vi "4_1_2.vi"() -> ()   [LabVIEW 2023, in "2025.lvlib"]
uses:
  2025.lvlib
  Program Files/National Instruments/LabVIEW 2025/user.lib/_OpenG.lib/lvdata/lvdata.llb/openg_variant.lvlib
panel:
  out "Intensity Graph":i32[][](graph)
  out "Array 3":i32[][](array[numeric])
  in  "Boolean":bool
  out "Result":i32
  out "Array 2":i32[](array[numeric])
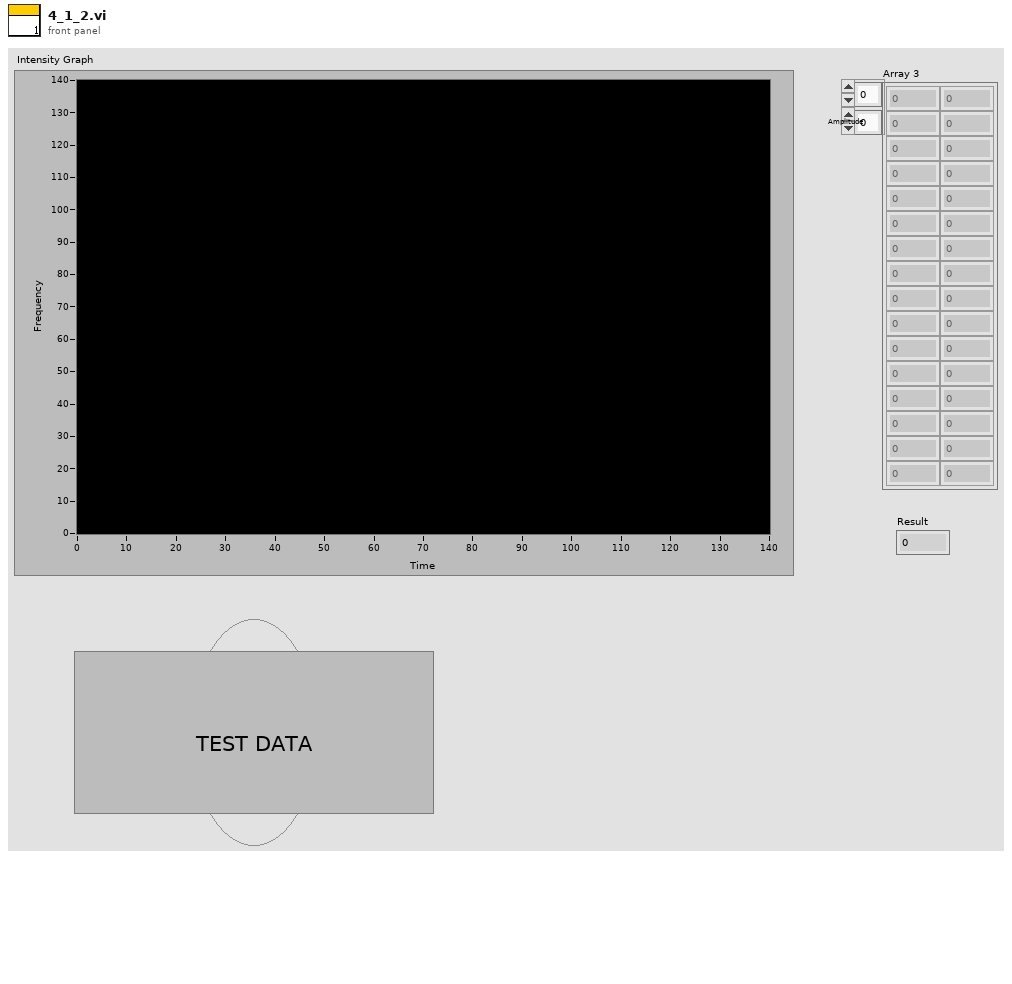
[diagram p1: front panel]
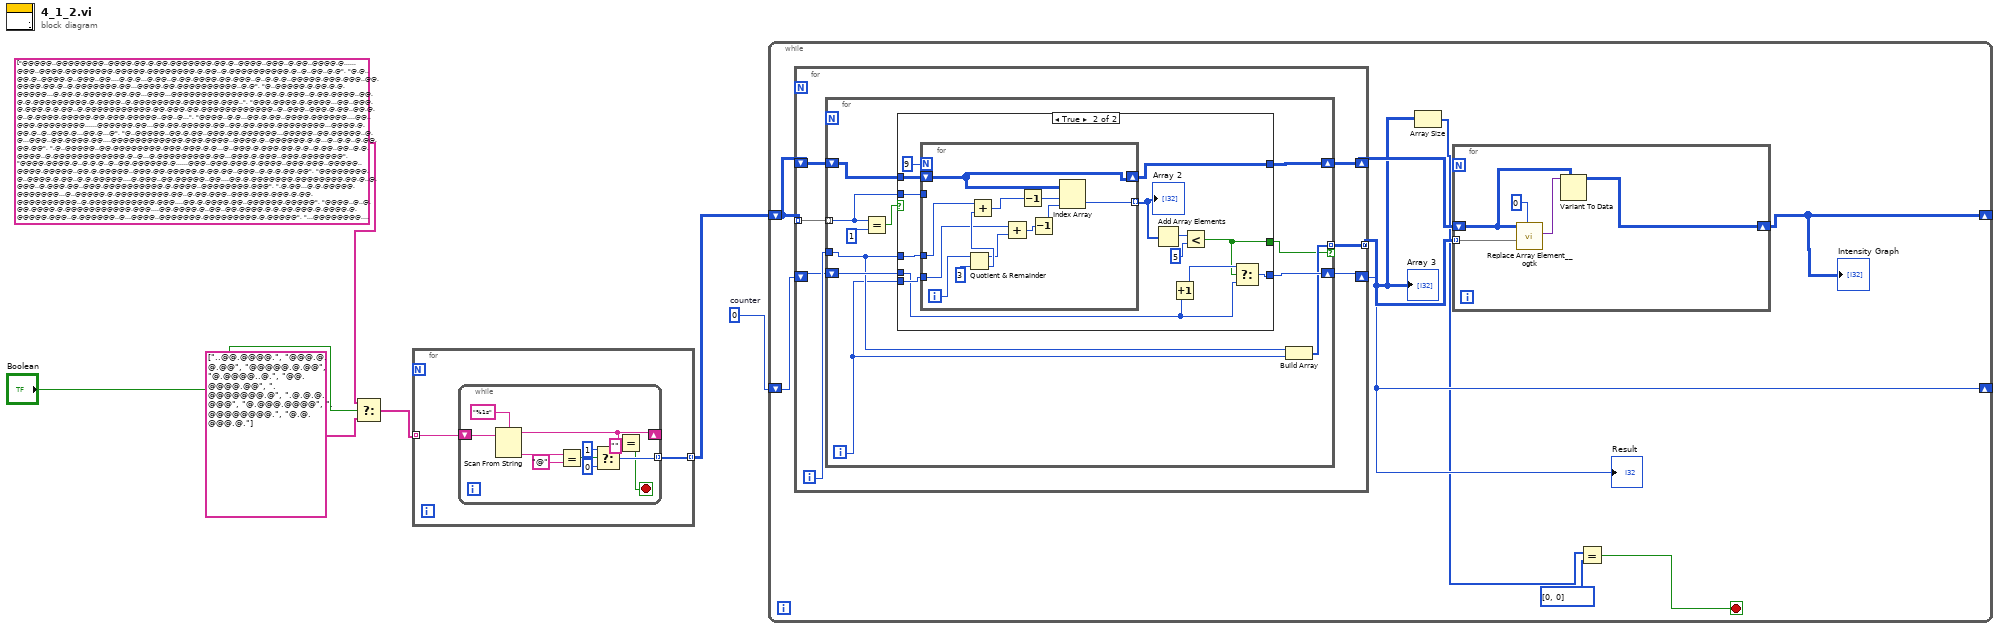
[diagram p0: block diagram]
diagram:
  w5 = 0  # counter
  n1 = Select(t=string[] ["@@@@@..@@@@@@@@..@@@@.@@.@.@@.@@@@@@@.@@.@..@@@@..@@@..@.@@..@@@@.@......@@@..@@@@.@@@@@@@@.@@@@@.@@@@@@@@.@.@@..@.@@@@@@@@@@.@..@..@@..@.@", "@.@..@@.@..@@@@.@..@@@..@@....@.@.@...@.@@..@.@@.@@@@.@@.@@@..@..@.@.@..@@@@@.@@@.@@@..@@.@@@@.@@.@..@.@@@@@@@.@@...@@@@.@@.@@@@@@@@@@..@.@", "@..@@@@@.@.@@.@.@.@@@@@...@.@@.@.@@@@@.@@.@@...@@@...@@@@@@@@@@@@@@.@.@@.@.@@@..@.@@.@@@@..@@.@.@.@@@@@@@@@.@.@@@@..@.@@@@@@@@.@@@@@@.@@@..", "@@@.@@@@.@.@@@@...@@..@@@.@.@@@.@.@.@@..@.@@@@@@@@@@@.@@.@@@.@@.@@@@@@@@@@@@..@..@@@..@@@.@.@@..@@.@.@..@.@@@@.@@@@@.@@.@@@.@@@@@..@@..@...", "@@@@..@.@...@@.@.@@..@@@@.@@@@@@....@@..@@@.@@@@@@@@......@@@@@@.@@...@@.@@.@@@@@.@@..@@.@@.@@@.@@@@@@@@...@@@@.@.@@.@..@..@@@.@...@@.@...@", "@..@@@@@..@@.@.@@..@@@.@@.@@@@@@...@@@@@..@@.@@@@@..@.@...@@@..@@.@@@@.@@....@@@@@@@@@@@@.@@@.@@@@..@@@@.@..@@@@@@.@.@...@..@.@..@.@@.@@.@@", ".@..@@@@@..@@.@@@@@@@@.@@@.@@@.@.@...@..@@@.@.@@@.@@.@.@..@.@@..@@..@.@.@@@@..@.@@@@@@@@@@@@.@..@...@.@@@@@@@@@.@@...@@@.@.@@@..@@@.@@@@@@@", "@@@@.@@@@.@..@.@.@..@..@@.@@@@@@.@......@@@..@@@.@@@.@.@@@@..@@@.@@@..@@@@@..@@@@.@@@@@..@@.@.@@@@@..@@@.@@.@@@@@.@.@@.@@..@@@..@.@.@.@@.@@", "@@@@@@@@.@..@@@@.@.@@..@.@.@@@@@....@.@@@..@@.@@@@@..@@....@@.@.@@@@@@@.@@@@@@@@.@@.@..@.@@@..@.@@@.@@..@@@.@@@@@@@@@@.@.@@@@..@@@@@@@@.@@@", ".@.@@...@.@.@@@@@.@@@@@@@...@..@@@@@.@.@@@@@@@@@.@@..@.@@.@@@..@@@.@@@.@@@.@.@@.@@@@@@@@@@..@.@@@@@@@@@@@.@@@....@@.@.@@@@.@@..@@@@@@.@@@@@", "@@@@..@..@.@@.@@@@.@.@@@@@@@@@@@.@@@....@@.@@@@.@..@@..@@.@@@@.@.@.@@.@@@.@.@@@@.@.@@@@@.@@@..@.@@@@@@..@...@@@@..@@@@@@@.@@@@@@@@@.@.@@@@@", "...@@@@@@@@.@@@@...@@.@..@@@@@@@@@.@@@.@@@@.@@.@@....@@...@@@.@.@.@@@@@@@@@@.@@.@.@.@@@.@@..@@..@@.@.@.@.@.@.@@@@.@..@.@..@@@@.@.@@@@@.@@@.", "@@@...@@@@@..@.@.@...@@..@.@@@@..@@@@...@@@@.@@@@@.@@@@.@@@@@..@.@@@@@.@@@@.@@@.@@@@..@@@@@..@.@@@...@@...@@@@@@@@.@.@@@..@@.@@@.....@@.@@@", ".@@@@@.@@@@@@@..@@.@@@@@@@@@@.@@.@@.@@@@@.@@@@@..@@@@@@@@@..@@@@@@@@@.@@@..@.@.@@....@@..@..@.@@@.@@@@@@...@@@@@@@@@@@.@.@@..@.@@.@@@@.@@..", "..@@@@@@@@@@.@.@@@@@@.@..@@.@.@@@@@@@@.@.@@@@@@@@.@.@@@.@@@@.@@@..@@..@@@@@.@@@.@@@@@@.@@@..@@@@@...@@@.@@@.@.@@...@@.@@@.@@@@@@@@@@@@@@@@@", "@@.@..@@@.@@@.@@@@@@@@@@@..@..@.@@.@@@.@@@@@@@.@..@..@@@..@@@...@..@@@@@...@@.@@@@@@@@...@@..@@.@@@@....@@@@.....@.@...@@@..@@@@.@@@.@@@@@@", "@@..@@.@@@.@@@@..@.@@@.@@.@@@@@@.@..@@@@@...@@@@@@@..@.....@@.@@.@..@@@..@@@@.@@@..@.@.@@@@.@@@@@@@@@@@@@@@@.@@.@.@.@@@@.@@..@.@@...@..@.@@", "@@@.@@@@@@@@@@.@@@@.@@@@@@@@.@@@@@.@@@.@@..@.@@..@@@@@..@.@.....@.@@@@@..@.@@@.@@@@.@..@..@..@@@...@@@@..@.@.@@@@.@...@@@@@@@...@..@@.@@.@.", "@.@@...@@.@@@@@@@..@.@.@@@..@@.@.@@@@...@.@@@@@@@@@@@@@@@..@@@@.@@....@@@@@...@@.@@.@@@@@@.@@.@@.@@.@@.@@.@@@.@.@.@@@@.@@.@.@@..@@..@.@@@@@", "@@@@.@.@.@@@@@@@..@@@@@..@@.@.@@@.@@@.@.@@@@@@@@@@@@@@@@@...@@@....@.@.@@@@@@.@....@..@@.@@@@@..@@.@@@@@.@@@@.@@@@@..@@@@@.@@@@.@.@.@@@..@.", "@@@.@@.@@@.@@@@.@@.@@@.@..@@.@..@@@@@.....@.@@.@.@@.@@.@@@.@.@@@.@@.@@@@..@..@@@..@@@@@.@....@@..@.@@@@@.@.@@@@..@@@@@@@@.@@....@@.@@.@@@..", ".@@.@@.@@..@@@.@@@@@@@.@@@.@@@@@@@..@@.@@@.@@@@.@@.@..@@@.@@.....@.@@...@@.@.@@.@@@@@@@@.@@..@@@.@.@.@@.@@@@@@@.@..@@@@.@@@@@@@@..@..@@.@..", "@@@...@@@.@@@@.@.@@.@@..@@@@@@@@@@@@.@.@@.@..@@@@@.@@@...@@@.@@.@.@.@......@@.@@.@.@@@.@@@@@..@@.@.@@..@@@@@@@.@@@..@..@@...@@@@@@@@@@@@@.@", "@@@@.@....@@@@@@@@@@@..@@..@.@@..@@@@.@@@@@.@.@@@.@.@@.@@@@@@@@.@...@@.@@.@@@.@@@.@..@@.@@.@@..@@.@...@@@.@.@@@...@@@.@@@@@@@@.@.@@.@..@@@@", "@@@@.@.@.@@@@@@@@.@@@@@.@.@.@.@.@@.@@@.@@@.....@@.@.@.@@@.....@@..@.@@@@@.@...@@@@@@.@@@.@.@..@@.@@@@@...@@@@.@.@.@..@@@..@@@@@@.@@.@@@.@..", "..@@@.@.@@@@@@@@..@@@..@@@@@@@@@@.@.@@@@@@@@@..@@@@...@@@@.@..@@..@@@@.@@@@.@@@.@@.@@@@....@.@.@..@.@.@@..@@.@@@@@@.@...@@.@@@.@..@@@@.@.@@", "..@@@@@.@.@@@.@@..@.@..@.@@@@@@@@@.@...@..@@@@@.@@@@@.@...@@....@@@@@.@.@@.@.@.@.@.@.@@@@@@...@@..@...@@@@.@@@@.@.@..@.@@@@@@@@@@.@@@@.@.@@", ".@@@@@..@@@@.@@@@@..@@@.@@.@..@...@@@..@@@@@.@@.@@..@@@.@@..@@...@@@.@.@...@@.@@@@@..@@@@@.@@@@@@.@.@@@@.@.@.@.@@@@@.@@@@...@@@@@.@@@@@@.@.", "@@@.@@..@...@@@@@@..@@@@@@@...@@@@@@@@......@@.@@.@@.@.@.@.@@..@@..@@.@.@.@@.@@@.@@@@@@@@@@@.@@.@@..@@@@...@@@@@@@@.@.@@@.@.@@@..@@@@@@...@", "@..@@..@@@@@.@@@@.@.@@@.@..@.@.@.@.@@@.....@@@.@.@.@@.@@.@@..@@@@@@@@@...@@....@.@.@@@..@@..@@@@@...@@@@@@@@@@@@@@@@@@@.@...@@@@..@.@.@@@@@", "@@..@.@@@.@@@..@.@@.@@@@@@..@@.@..@@@@@@.@@@.@@@...@@.@.@@@@.@.@@@@@..@@@@@@.@@@@.@.@@@@@@@@@@..@@.@@.@@.@@@.@.@@@..@@.@@.@@.@.@@@@@@@..@..", "@..@@.@..@@@@@@@.@.@...@.@@@@@@.@@@@@....@@@@@....@@@.@@..@@@@..@@@.@.@@@@@@@@.@..@@@@@..@@@@@@@@.@@@.@@@@@@@@.@@@@.@@..@@...@@@@@.@@@.@@@.", "@@@@@@@..@@@.@..@.@..@@.@.@@@@.@@@@.....@@.@.@@@.@@..@@.@@@.@..@@.@.@@.@.@.@@.@@@.@@.@@.@@@@@.@..@@.@...@@.@..@@@@@@@@@..@@@@@.@@.@@..@.@.@", "@.@@@.@.@.@@.@@@@.@@....@@@@@.@@@..@..@@....@.@@@@@@..@@@.@@@@@@..@.@.@@@....@.@...@@@.@@@@@.@.@.@@@@@..@@@.@.@@..@@.@.@.@@@@@@.@.@..@@.@.@", ".@@..@@.@.@@@@@.@@.@..@@.@@.@@@@@@@@...@.@@@@@@..@@@@@.@@.@.......@@.@@@@@@.@.@.@.@@@.@.@@@.@..@.@@@@...@@@@.@@..@..@@@@@.@@@@@.@@@@@@@@@@@", "@@@@@@@@@.@...@@..@.@@@@@.@@@..@@@@@..@@@@.@.@.@.@@@@@@@@@@@@.@...@.@@@@@.@@.@@@@@@.@@@@@@@.@..@@@@.@.@@@@@@@@..@.@@@@@@@.@@.@@..@@@@@@@@@@", "@@@...@@@@@@@.@@@@@@..@.@@@.@@@.@..@@.@@.@@.@@.@.@@.@.@@@..@@@@@....@@@@.@..@@...@@@@@@.@.@@.@@@..@.@.@.@@@@.@@@...@@@@@@.@@@..@.@@.@@.....", "@@.@@@@@.@.@@@@...@@@@@@@.@.@@....@@.@.@@.@...@@.@@@@@@......@.@@@@@...@.@...@@@@@@@.@@..@@@.@@@@@.@.@@.@@@@..@@.@.@@@@@@.@@...@@..@@@@@.@@", "@@@.@@@.@@..@@@@....@.@.@.@.@@@@.@..@@@@.@@@@@@@@@@..@.....@.@@.@@@.@@@@@@.@.@@.@@.@.@@@@@.@@@@@@@..@@@@@.@...@@@..@....@.@@@.@@.....@..@.@", "@@@.@@.@@@@..@@@.@.@@.@..@@@@.@@.@@@.@@.@@.@@@..@@.@..@@@.@.@@@@..@.@@@@@.@..@@.@.@@@@@@.@@@@@.@.@@.@@@@.@@@..@.@@.@@.@.@..@@@.@.@@@.@@.@@@", "@.@@@@@@@@..@@@@@@@@@@..@@@@.@@....@.@...@@@@....@@@@.@@@@.@@@@@@.@@.@..@.@@@@@.@.@@@@@..@@.@@..@@@.@@.@.@@.....@@@..@@@@..@@@@@.@@.@@@@..@", "..@@@@@@@@@.@@@.@@@@@.@@@..@.@...@........@@@.@@.@@@@@...@.@.@@.@..@..@@@.@.@...@@@.@.@@.@..@@@@..@@@@.@......@@.@@..@.@@..@@@..@.....@@@.@", ".@@@@..@.@@.@@@.@@@@@@@.@@@..@@..@@@.@..@..@@@.....@@.@@@@@@@@.@.@.@.@@@@@@..@@@@@@.@@.....@.@..@@..@@..@@@.@@@@.@@@.@@.@@@.@.@@..@@.@@@..@", ".@@@@@@@@@@@@@.@@@@.@..@@.@..@@.@@.@.@@.@@@@@@@.@@.@@@...@@@.@@..@@..@.@..@@@@@@@@@@@@.....@@@@@@@@@@@@.@@.@@.@@@.@@.@....@@@...@@.@.@@.@@.", ".@....@@@@@@@@@@..@@.@@@@..@@@@@.@@@@@@..@...@.@.....@@@@@@...@@.@@.....@@@@@@@.@@@@.@@.@.@@@.@@.@@@@@@@@@..@@.@.@@@.@@@.@@@@.@@.@.@..@.@.@", "@@@@.@@.@..@@.@@@@@@@..@.@.@..@..@@@.@@@@@@@.@.@.@@@..@@@@@@.@@@.@.@..@@@@@@@@@....@@.@@@@@@..@@@..@.@@@@@..@@....@@@@@@.@..@@@...@.@.@..@@", "@@.@@@@...@@.@.@@.@@@.@@@@@....@@@@@@.@@.@..@.@.@@.@@@@.@.@@@@@@..@@@...@@@@@@@....@.@@@@.@@@@@.@@@.@@..@@.@.@..@@@@@@@.@..@@@@@@@@..@@.@@@", ".@@@@.@@@@.@.@...@.@@@..@..@@@@@@@@.@.@..@.@..@@@@@.@..@@@@@@.@@@@@@@.@@@.@@@...@.@.@@@@@@.@@@...@.@..@@@@@.@..@..@.@..@@@@@@@@@@.@@@.@.@@.", "@...@.@@@@@.@@@@@..@@.@@@.@@@@@..@@@@@@@@@@@...@@@@@@.....@@.@.@.@@@@@@@@..@@@@@@@@@@@@.@.....@@.@..@@@@.@...@@@@@@@@...@@@.@@@@.@@@@@@@...", ".@.@..........@...@....@...@@.@@@@@@@.@@.@...@@.@..@@..@@@..@@@@...@@...@@@..@@..@@@@@.@@@@@@@.@...@@@@@@@@@@..@..@@@@@@.@.@@@@..@.@@@@@.@.", "@@.@@@@.@@.@@@@.@@.@@@@.@@@.@.@@.@@@@@.@@@.@..@@@@@.@@@..@@..@@.@.@@...@@@....@@..@@..@.@@@...@@@@.@@...@..@@@@@..@@@@@@.@@.@.@@..@@.@.@@@@", "@@@@@....@....@@.@..@@@@...@...@@.@.@@@..@@@@.@..@.@@@@.@@@@..@.@.@.@@@@@..@@@@.@@....@.@.@.@..@..@@.@..@@@@@.@@@.@@@@@@@@.@@@@@@.@@@@.@@.@", "@.@....@..@@@@@@@.@@@.@.@@@@@.@.@@@.@@@@@@@@.@@@.@@@.@@@@.@.@..@.@@@@@@..@@.@..@@@.@.@@@@.@@@.@@@@..@@@@.@@@@@..@@@.@..@@@@.@.@@@@.@@@.@...", "..@@@@@@@@...@@@@.@@.@@@..@@@@..@@.@@.@..@......@...@@....@@.@@@@@@.@@@@@@@@@@@..@@@.@.@@@@.@..@@.@.@@.@..@.@@@@@..@..@@@@@@.@.@.@.@@.@@@@@", "@.@....@.@@...@@@@@@.@@@@@.@@@@@@@@.@.@...@.@.@@@.@@@@@@......@...@.@@..@@.@@@@.....@@@@@@@...@@...@@@.@@.@@@@@@@@@@@@@.@@@@@@@.@@@@@@.@@@@", "@@@@.@@@@@@..@@.@@..@@.@..@.@..@@@@@@@@@@@....@.......@..@.@@.@@.@@@@@@@@@@.@@@@@@@..@..@@.@@@.@@.@.@@.@...@..@..@@@.@.@@@..@@@.@..@.@@@.@@", "@@@.@@.@@@..@@@.@@.@@.@@.@@@@@@@@@.@.@.@@@.@@.@@@...@@.@@....@@@@.@@..@@@@@@.@@@.@@@@@.@@....@@@@@@.@...@@.@.@@@.@@@@.@@@@...@@@@@@@.@@.@@@", "@.@@@@..@.@...@@@@@@@@@..@@@@@@@@@@@.@..@@@@@.@....@.@.@@@.@@.@...@.@.@@@@...@@@...@..@@@@@@@@@.@.@@..@@@@@@.@@.@...@@..@@.@@.@@@.@..@.@.@@", ".@@@.@.@@...@.@@@@@@@@@@.@@@@.@.@.@@@@@.@.@@@@@@@@@@@.@.@@@@@@@@@.@...@@@@.@@@@@.@...@@.@@.@@@@..@@@@@@@.@@@..@@@.@@.@@@@@.@@@@@@.@@@@@@..@", "@.@@.@@.@@@.@@@@@@.@@.@@.@.@@@.@@..@@.@.@@@@@.@@@@....@.@...@@@@.@.@..@@@.@@@.@.@.@.@.@...@.@@.@@@@.@@.@@..@.@@@@@@@.@.@..@.@@.@.@.@@.@@@@.", ".@@..@..@@@@@@@@.@@@@@.@.@.@.@@@@@....@@..@@.@.@.@@@@@@.@..@..@.@@..@@@@@@.@..@.@@.@@@.@..@..@.@@.@@@@@@@.@@.@@@@.@..@.@@.@@@.@@.@@@.@.@..@", ".@@.@@@.@@....@@..@.@.@.@@@..@.@@@.@@@@@@.@@@@.@@@.@@.@@...@.@.@@@@@@..@..@.@.@@@@@@@@@...@@@..@.@..@..@@.@@@..@..@@@.@.@@@@@...@@@@@@@@@.@", "@@.@..@@@.@@...@@@@@..@@....@@@@@@@@@.@.@@@@.@...@.@@@..@@@@@@@@..@@@.@@..@.@@@..@@@@.@@@..@@@.....@...@.@.@..@.@.@@@@...@@@@.@@@@.@.@@@..@", "@@@@@.@@..@@@@.@@.@@.@.@@@@.@.@@@@@@.@@..@@..@@@...@.@@@@....@@.@.@..@.@@@...@@.@.@@@@@@@@.@.@@.@.@@.@@@@@..@@.@@@@@@@@..@.@@@@.@@.@@..@..@", "@@.....@@@@.@@.@.@@@@@@@@.@@@@@..@.@@...@.@@.@@@@@@@..@@.@@.@@@.@.@@.@@@@.@@@....@@@@..@@@.@.@..@@....@@@..@....@@.@.@..@.@@@@@@@@.@@@..@@.", ".@.@@@@..@@@.@@.@.@@@.@@@@..@@@@@@@@@.@@@@.@@@@.@@@.@@@.@@@...@..@.@@...@@@@@..@@@.@@@..@@.@@@@.@@.@@@.@@@@@@@@.@.@...@.@.@@..@.@@@@..@@@@@", "@@..@.@.@@.@@@@@@@..@@@@.@@.@@@@..@@@.@@.@@@..@@@@.@.@@.@@@@.@@.@@@@@@@@@.@.@...@@@...@@@.@@...@@@@.@@.@@..@.@...@@@@@@@.@@@.@@@...@@@@.@@@", "..@.@@@@@@..@@..@.@@@@.@..@@@@....@....@.@@.@@.@..@.@@.@.@@@@@.@@@.@@@.@@@@@.@@@@.@@...@@@......@@.@@@.@.@@.@.@@@@@@@@.@@@.@@@@@@@@@@.@.@@.", "@.@..@..@.@@@.@.@.@.@@@..@@..@@..@....@@@@@@.@@@@...@.@.@.@@@@@.@@@@@@@@@.@....@.@..@@@.@@@@.@@@.@@.@@@@@@.@@.@@@@@@@.@@@..@...@@@..@@...@@", ".@@@@@...@@.@.@@@@@@@@@@@@.@@@..@.@.@@@..@.@..@@..@.@@@.@@@@..@..@..@@.@.@@..@..@@.@...@@@@@@@.@@@@.@@..@.@@@@@@@@@.@@.@@@.@@.@@.@..@@@@@@@", "..@..@@@..@.....@.@@@@@@@@@@@.@.....@.@...@.@@@@@@@@@@@..@.@@@@..@.....@@.@.@@@@@@.@@@@..@.@.@@@@@@@@@...@.@@@.@@...@@.@.@@.@@...@@@@@@@@@@", "@...@@@.@.@@@.@.@@@..@...@@@@@@..@@.@.@@.@.@.@@...@.....@.@@@.@...@@@..@@@@@...@.@@.@.@@@.@@.@@@@@@.@@@@@@@@@.@@@@@.@.@@@..@.@@@@...@@@@@..", "@@@@@@.@@@.@....@.@.@.@@@@.@@.....@@.@..@..@@@@@@...@@..@@..@@@@@@@.@..@@.@..@.@@@@@@@@@..@.@@@.@@@.@@.@@@.@@@@...@......@.@@@.@@@@.@@@.@..", "@@@@.@@@...@@@@@@..@@.@.@@..@@@.@@.@@@...@......@@@.@@@@@@....@@@.@@.@@@@.@...@@@@@@@@.@@..@@.@@@@.@@@.@.@@@@@.@.@@.@.@...@@.@@@.@@@@@@@@@.", "...@@.@@@@....@@..@.....@@.@@...@@@..@.@@.@@.@@@.@@@.@@@@.@@.@@@@.@@..@.@@.@..@@@@@@.@@@@@@@..@@@@@@.@@@@@@.@@@@@.@...@@@..@.@@@@@@@.@@@@@@", "@@.@.@.@.@.@@@@@@@@@@......@@@@@@@@@.@@..@@@@@@@@@@@.@@.@@@.@.@@....@.@..@@..@@@@..@@@....@@@..@.@@..@.@@@..@@.@.@@@...@@@@@@@@..@@.@@@....", "@@@@.@@@@@@@@@@@@@@@@@@@.@@.@@@@.@@@@.@@..@@.@@@@.@@.@@@@.@.@@.@.@@@@.@@.@@@@@...@...@@.@.@@@@...@@.@@.@@@...@.@...@.@@.@.@@.@@@@.@@@@@@@.@", ".@.@.@@@@@@@@@..@@.@@@@..@.@@.@@.@..@@..@@@@.@@@..@@@...@@@@.@.@@...@.@@@@@@@..@.@@.@@@@@.@@@@@@..@@@@..@@@@...@@....@@@@.@.@@@.@@..@.@@.@.", "@@..@.@.@.@@@@@@.@@..@..@.@.@@@@@....@@@@.@@@@@@.@.@.@@..@@...@@.@..@@@.@.@@.@@@@@.@@.......@.@.@.@@..@.....@@.@@.@@@@..@@@.@.@@@@@.@@@.@@@", ".@@@..@..@@@@..@@@@@@.@...@.@..@@@.@@@.@@.@@@..@@@@.@@@@.@@....@@@.@@@@@@@@.@@@@.@@.@@@@@@@@@......@@.@@.@@@@.@.@@@@.@..@@.@.@.@@@@.@@@@@@.", ".@@@@@@....@@.@..@.@@@@.@@@@@.@@@.@@@@.@@@@@@@@..@.@@@@.@@@@@@@@@@@@@..@@@@@@.@@@@@.@@.@@@@@@@@.@.@@.@@@@@.@@.@.@@@@@@@.@@@@@@.@.@@.@.@@@.@", "@@@@@...@@.@.@.@.@@@.@.@@@@.@..@....@@@@@@@.@...@@.@@..@@@..@@.@@@....@@@@@.@@.@.@..@..@@@.@@...@.@@@@@@.@@@@@@@..@...@.@.@.@.@@..@.@@@@@..", "....@@@@.@.@@..@@.@@.@@.@@@@@..@@.@.@@.@@@..@@.@.@@...@.@.@.@@.@@@@@@.@@@@@.@.@.@..@@@@@@.@@@.@@@.@.@@@@..@..@@.@@@..@@@@..@.@@@@@@@@@@.@@.", "..@@.@@@@.@.@@@..@@...@@@@@@@.@..@@.@.@.@@@@@@.@@.@@@.@@.@@@@@..@.@@@...@@@@@.@@.@@.@@..@@@@@@...@@..@@...@@@@@@@@@@@@.@@.@@@@@@.@@.@@@@..@", "@@@..@@.@@@@@...@...@@@@@.@@...@.@@@@..@@.@.@.@.@@.@@@@@@@..@@@@.@@@@.@@@@@..@@.@.@.@.@@@.@..@.@@@@@@@@@@.@.@.@@@@@@@@@.@@@@@.@@.@.@@@.@.@.", "@@@.@@..@...@@.@.@@@.@@.@@@@.@@@@@...@@..@@@@.@..@@.@@@@..@@@.@.@.@..@@.@@@@@@.@.@@@.@@.@@@@@.@@@@@@@@.@...@@.@@@@.@.@@@.@@@@..@@@@@.@@..@@", "@@...@@.@.@@.@@@.@..@.@@@@@.@.@@@.@@@@@@.@@.@.@@@@@.@@@@@.@@@@@@.@@@@....@..@....@@@..@.@.@@@@@.@@@@@@@@@@@.@@@@@@@@.@@.@@..@..@@@@@..@..@@", "@..@@@.@.@.@@.@@@.@@@@@.@@@.@@@@.@@.@.@@.@@@@@@@.@@@...@@.@@@@@@.@@@.@..@@@@@@.@@....@.@@@@@@@..@..@@.@@@.@@@@@.@@@@.@@@@@.@.@@@.@.@.@.@.@.", "@@@.@@..@@@@.@.@..@@.@@..@@..@@.@.@@.@.@@.@..@@@.@@@@.@..@.@..@@@@@@@.@@@@@@@@@@..@@@.@@.@@..@.@..@.@@@@@@@.@@@.@.@@@.@.....@.@..@@@@@@...@", "@..@.@..@@@@@...@@...@..@@..@@.@..@@@@.@..@@..@@@@..@@@.@@...@.@@@@@@@@....@@@.@@@@@@@@@@@@@.....@@..@@@@@@@@@@.@@@@@@@@.@@@@@@...@@..@@@@.", "@.@@.@.@.@.@..@@@.@@...@@@..@.@@.@@@@@......@@@@@.@@.@@@@@@..@@...@...@..@@.@@.@@..@@.@@.@@.@@.@@@@@@.@@@..@@.@@@@@@@@@.@.@.@@@@.@@@@@@.@@@", "..@@@@@@.@...@..@@@@@@@@@.@@@@@...@@@@@@@@@@@@.@.@@..@.@@@....@@@.@..@@@@@@@@@@.@@.@@@@.@.@@.@.@@@@@@.@@@@..@.@@@..@@@@.@@@@@@@@@..@@@@@.@@", "@@@@@@.@@@.@@.@..@@.@..@.@.@.@@.@@@@@@...@..@@.@.@@@@.@.@@@..@.@@..@.@@@...@@@...@.@.@@.....@@.@..@@@@.@@..@@.@@@@@@@..@.....@@@.@.@@@@..@@", ".@@....@.@.....@.@@@@....@@@..@...@@@@@@.@@@@.@@@.@@.@@@..@@.@@@.@.@...@@@.@.@@.@.@.@@@..@@@@@.@@@@@@@@@.@@.@.@@.@.@@.@@..@.@@@@.@@@@@@@@@@", "@.@@@@@@@.@@@@@.@..@@@@@@.....@..@@@@@.@@@.@@@.@@@@.@..@@.@@@..@@@.@@@@@.@@@@@@.@@..@@.@..@@@@@@@@@@@@.@@.@@.@@@..@@.@@@@..@@.@@@@@@@@@.@..", "@@.@@.@.@@@@..@@@@.@@@@@@@@...@@@@..@@..@.@@.@@@@@@@@.@.@@@@.@@@..@@@@@@.@@@@@.@@.@@.@....@@@@@@..@@@@.@@@@.....@@...@@.@@.@@@.@@@@.@@@.@.@", ".@@@.@@@@@@.@.@.@@@.@.@.@..@@.@.@@@.@@@@@@@@@..@@.@.@@@@@@@@.@.@.@.@@.@@..@@...@.@@@@@@@.@.@@.@.@@.@..@@@..@@.@.@@@.@@..@@@@@@@@.@@@@@.@@@@", ".@@.@@@.@@@.@@@..@@.@@..@@..@@@.@.@@....@@..@..@@@@@@@@@@@.@@@.@.@@@@..@@.@.@@@@@@@@@..@.@.@@@@@@...@@@@.@..@@.@.@.@@@@@.@..@@@@@@..@...@@@", ".@@@@.@@@@@@@@.@@.@@@@@..@@@@.@.@@@...@@@.@@@..@@@@@@@@.@.@@@.@@.@@@.@@@@@@@@@.@..@.@.@@..@@@@...@@..@@.@..@.@@@@..@@@@@@..@@@....@.@@@@.@@", ".@@.@..@.@..@.@@@@@@@@.@@@@@@@@@@..@@...@..@@.@@.@@@.@..@..@@.@@@@@@.@.@.@@.@@@.@@...@@@@@@@@@..@@@@@...@.@@@@..@@@.@.@.@.@@@@..@@@@@.@@..@", "@@@.@@@.@.@@.@@@@.@.@@@.@@@@@@.@@@@.....@@@@@..@@@...@.@@@..@@@@.@@..@@@.@@@..@@@@..@@.@@.@..@@.@@..@.@@@@@.@@@@.@@....@@@@@@@@.@@@@@.@.@..", "@@...@@@@@@@@@@@@@..@.@@@..@@@@@@@@@@.@@.@..@.@@@@...@.@..@@@.@@.@.@.@@@@@@@.@..@@.@@..@@@@@@@@@@@.@.@@@@@.@@@@@.@@@@..@@..@.@@@@.@@@@@...@", ".@@@@.@..@@@.@@@.@@@@...@@@.@@@....@@.@@@@@@@..@.@.....@.@@@...@@@@@@@..@@@.@.@@@@.@..@@@.@.@.@@@@@@@..@@@@@..@.@@@@.@@@@@.@.@@.@@.@@@@.@..", "@@@..@@@@.@@@@..@@..@@@@@..@.@.@.@...@.@@.@@@..@@.@.@@@@@@@.@@@@...@@..@@..@@@.@..@@@.@.@@@@.@.@@@@@@@@.....@@.@@@@@..@@@@@@....@@@.@@@@@@.", "@@.@@@@@@@@@..@@@.@.@.@..@..@.@..@@@..@@..@.@@@@.@@@@@@@@@@@@@@@.@..@@@@@@@@@@@@.@@@@.@@...@@@.@@.@@.@@@@@@.@@@@..@...@.@@@@@.@.@.@@@@@@@@.", ".@.@@@.@@.@@..@@.@.@...@.@.@@..@..@@@..@@@@.@@@..@@@..@.@.@.@.@@@@@@@@@@....@@.@@@@.@@@@@@..@@@..@@@.@@@@..@..@@@.@@@@@@@.@.@.@@@@@@@@...@.", ".@....@.@.@@@@@.@@@@.@@@.@..@...@@@.@@.@@..@.@@@@@@@@.@.@.@@.@.@@..@@..@.@...@@@@@.@@@@@..@@.@@@.@@@@..@@.@@@@@@.@....@@@@@@@@@@@.....@@.@@", "@..@@.@@@@@@@@@.@@@.@..@@@@.@@@@@.@.@@.@.@@@@@..@@@.@@.@@@..@.@.@@@...@.@.@@@..@@@@@@@@@..@.@@@@.@@.@@@@@@@@..@@.@.@@@....@@@@@@..@.@...@@@", ".@@@@@..@@@.@..@@@.@@@.@.@@.@@.@@.@...@.@.@@..@@@@@@@...@@..@@@@@@@.@@@..@..@.@@@..@@@@@@.@@@@..@.@@@@@@@@@@@@.@.@@.@@@.@@@.@@.@.@.@.@.@@@.", "@@@@@..@...@@@...@@@.@.@@@@...@..@@@@@@@@..@@...@.@.@@@@@.@@@@.@@@.@@@@@..@@@...@.@@@@@@@@.@@.@@@...@@@@@@.@@@@@.@@@@@@@.@@.@.@@.@@@..@@@@@", "@..@.@@.@@@@@.@@.@@...@@@.@@@....@...@..@..@.@@@@.@@@@@@@@@.@.@@@@@@@@..@@@@@@..@..@.@@..@@@.@@...@.@.@.@..@@..@@@@.@.@.@..@@.@@.@.@@@@@@@@", "@@.@.@.@@@@....@.@@@@.@@@..@.@@@.@.@@.@@..@@.@@@.@...@.@@@@@@@@@..@..@@@@@@@.@...@@@..@@@..@..@@..@@@@@@...@.@@.@@@@@..@@@@@@.@@@@@.@@@@@@.", "@@..@@@@@@.@..@.@.@@@@.@@@@@.@@@.@@@@@@@.@@@@@....@@.@@..@@@@@@@@@...@.@@@.@@@.@@.@@@@.@..@.@.@.@@@@@.@@@@...@.@@@@@@.@.@@.@@@@@..@@@@@.@@@", ".@..@@@.@..@.@.@...@@@@@.@@@@.@@@@@@@@@@@.@@.@@@@@.@@.@@.@@@.@@@.@...@.@@@@@@@.@.@@@@.@@@@@@@@@@@@...@@@@.@@.@@@@@@@.@@.@@@.@.@@.@@@.@@@@@@", "@@@@.@@@@.@@@@@@@@@@.@@@@@...@.@@@@@.@@@@@@@@@.@@@..@...@@...@@@.@..@@@..@.@@.@@@@.@@@@.@@@@@@@@@.@@@@@@.@@@.@.@@@.@@.@.@..@@@@.@..@@@..@@@", "....@..@@.@.@...@@@@@@..@@.@@.@@..@@@..@@..@@.@..@@@@.@@@.@@@@@.@@.@@..@..@@..@@@@@..@.@@@@@@@@..@.@@..@@@@..@@@@..@@...@...@.@..@@@@@@@@..", "@@..@@@@.@@.....@.@@@@..@.@@..@@@.@@@@@@@@@@@@@@.@@@@.@@@@.@@.@@.@@@@@.@@.@..@@.@......@@@.@@@..@@@@@@@@@@.@.@@...@@@@@@@@.@.@@.@@@@@.@@@@.", "@@@..@.@@.@@@@.....@@@.@.@@@.@@@.@....@@@@.@.@.@@@..@@@.@@.@@@.@@.@.@@..@@@@@.@.@@..@.@.@...@@@.@.@.@@@@.@@.@@@.@@..@..@@@.@.@@.@@..@..@@@.", "..@@.@@@@@@@@.@.@@..@..@@@..@..@@@..@.....@@@@..@@@.@@.@@@.@@@....@@.@.@@....@@@@@@.@@@.@@@.@@@.@@@.@@@@@@@.@@....@@@@..@.@....@@@@.@..@@@@", "@..@.@@.@@.@.@@@.....@.@@@@.@.@@.@@..@@@@.@..@@@@@@.@@@@@.@@@@..@@@@@@@@@@@@@.@.@.@@@.@.@@@@@@@@.@.@@@@.@@@.@@@@@.@@@@@@..@@@@@..@.@.@@@@@@", "@@@@@..@@@..@@@@@@.@@@.@.@.@@@..@@@@@@@.@@....@@@@@@@..@@..@..@@.@@@@@.@.@@@....@@@@@@.....@....@@.@@@@.@@@.@@@@.@@@@.@@@@@@..@@.@@...@@@.@", ".@....@@.@.@..@.@.@@@@@@@@@.@@.@@@.@...@.....@@.@@...@@@@@@@..@.@@@@@.@@.@@@@@@@.@@..@.@@@.@.@@@.@@@@@@.@@..@@@.@@..@@@.@@@.@.@@...@@@@..@.", "@..@@@@@@@@.@@@.@@@@.@..@.@@@.@@@@..@@.@@@@.@@.@@@.@@@@@@@@.@@@..@@..@@@@@.@@.@.@@.@.@@@.@@@.@@.@.@@@@....@@@..@.@@.@.@.@@@.@@@@@@@@@.@@@@@", ".@@@.@@@.@@@@.@.@@@@@@@.@.@@@@@@@.@@@@@@.@@.@@@.@@.@.@.@@@@@@...@@@@@.@@@@....@.@@@@@..@.@@@@@@@@@.@.@@.@.@@...@.@.....@@.@@@@@@@..@@@.@.@.", "@@@@..@@@.@@@.@@@@@@@@@.@@.@@..@.@@.@@...@@.@@@.@@.@@..@@..@@@@.@@.@@@@@@@@@.@.@@@@@@.@@@@..@..@@..@@@.@@.@@@@@@.@@@@.@.@.@@@@@@@@@....@@.@", "@@@.@@@@@@.@@....@@@@@@@@@@@@@@.@@@@@@.@@@@.@.@.@@@@.@@@..@@.@@...@@@@@.@@@@@..@....@@@....@@.@@.@...@.@@@.@@...@@.@@@@.@@@@.@..@.@@@@@@@..", "@@@.@@..@..@.@@@@.@@@@@@@.@@@@@.@..@@.@@@@.@@@@.@.@@.@.@@@.@@@..@@@..@@@@...@@.@@@@.@@@@@..@.@@@@@@.@@@.......@@@@.@@@@@..@@..@@@@@..@@@@@@", "@@.@@@@..@.@..@..@.@.@.@.@@@@@...@.@.@.@.@....@.@@.@@@.@.@@@@@@...@.@@@.@@@@@@@.@@@.@@@@.@....@@@.@.@@.@.@@@@@..@@@@@@....@@@..@@.@....@@@@", "@@.@@@@@@.@@.@@@.@.@@@.@..@@@..@@.@@.@@..@@@.@@@.@@..@@@@@@@.@@.@.@..@@@@@@@@.@@@@@...@@.@@@..@.@@@@@@.@@@...@.@.@.@@@..@.@@...@@@@..@@@@@.", ".@.@.@..@@@@@@@@.@.@@..@..@@..@@@.@.@.@@.@@.@@@@@@..@.@@.@..@.@@@.@.@@@.@@@@@.@.@@@@.@.@@...@.@@@..@@@@..@.@@@.@.@.@@..@@@@@@.@@@@..@.@@@@@", ".@@.@.@@@@@@.@..@@@@@@.@@@@.@.....@@@@@@.@@..@.@@@..@@..@@@@.@.@.@@.@..@.@@@@.@@@@@.@@..@@@.@..@...@@@@@@@..@@.@@@.@@@@@.@@.@.@@@@@.@@@@..@", "..@.@..@@.@@.@@@@@@@..@.@...@..@@@...@@@.@@@@....@@@@....@@@@@@@.@.@@.@@@@@@.@@.@@...@@@@..@.@..@.@@@@@.@@..@@@.@@@@..@@@.@@@@..@@.@.@..@@.", "@.@@@@@@@@@.@@@@..@.@.@@@@..@@..@@@@.@@@@@..@@...@@@@..@.@....@.@@.@.@@.@.@.@.@@@@@@.@@.@....@.@.@..@@@.@..@@@@.@@@@@.@.@.@@@.@.@.@.@..@@@@", "@.@@@@.@...@@@.@@..@.@@.@@@...@..@@.@@@@@@@@.@@@@@.@.@..@..@.@@@.@...@@@.@@..@.@..@.@@@...@@@@@@@@@@@@..@@@@@@..@@@..@@@.@.@@@..@@@@@.@.@@@", ".@@@@@@.@....@.@..@@@@@.@.@@.@@@.@@@@..@.@.@.@.@.@...@.@@.@@@@..@@@@@.@@.@..@@@@@@.@.@@@@@@@@@@@.@..@.@@..@.@@@@@@.@@@.@@.@@@@@.@.@..@.@@..", "@@.@@@.@.@@@@@..@.@@@@@@.@@.@.@@@..@@@@@@@.@@@@..@@@@@.@..@.@.@..@.@@@@@.@.@@.@.@@@@@@@...@..@.@.@@..@@..@@@@@.@.@@@@.@@..@@@...@.@.@.@@.@@", "@@@@@@@@.@..@.@@.@..@@@....@....@..@@@.@@@@.@@@..@@@@@@@..@.@@@@@.@.@@..@@@..@@.@@@@.@.@@@.@@.@@@@@@..@.@@.@..@.@@.@@.@@@@.@...@@@@....@@.@", ".@@@@@..@....@@@@...@@@.@.@.@@@@.@@..@.@@..@@@@..@.@@@@@@@@@.@..@.@@@@.@@@@@.@@@.@.@@@..@@...@.@.@..@@@.@@.@..@@.@@@.@@.@@.@@@@.@@..@@@@@@.", ".@@@..@@@@@@@....@@@@.@@@@@.@@@@@@@.@@@@@.@@.@@@@.@.@.@@.@@@@..@@.@......@@@@.@@@@....@@.@@@.@.@@.@@@@@@.@@@@@.@.@@...@@.@@.@...@@@..@@@@.."], s="Boolean", f=string[] ["..@@.@@@@.", "@@@.@.@.@@", "@@@@@.@.@@", "@.@@@@..@.", "@@.@@@@.@@", ".@@@@@@@.@", ".@.@.@.@@@", "@.@@@.@@@@", ".@@@@@@@@.", "@.@.@@@.@."]) -> (s? t:f=w2:string[])
  n2 = for {
    tunnel: w2 -> [w8] mode=indexing
    tunnel: [w7] -> w6 mode=indexing
    n3 = while {
      shift-right: [w11] -> _
      shift-left: w8 -> [w19]
      tunnel: [w12] -> w7 mode=indexing
      stop <- w9 stop-if-true
      n4 = Scan From String(format string="%1s", input string=w19) -> (remaining string=w11:string, output 1=w17:string)  [unwired: 3 in, 2 out]
      n5 = Equal?(x=w17, y="@") -> (x = y?=w15:bool)
      n6 = Select(t=1, s=w15, f=0) -> (s? t:f=w12:i32)
      n7 = Equal?(x=w11, y="") -> (x = y?=w9:bool)
    }
  }
  n8 = while {
    shift-right: [w20] -> _
    shift-left: w6 -> [w28]
    shift-right: [w24] -> _
    shift-left: w5 -> [w27]
    stop <- w21 stop-if-true
    n9 = for {
      tunnel: w28 -> [w40] mode=indexing
      shift-right: [w38] -> w26
      shift-left: w28 -> [w39]
      shift-right: [w35] -> w24
      shift-left: w27 -> [w36]
      tunnel: [w34] -> w25 mode=concatenating
      i -> [w37]
      n10 = for {
        tunnel: w40 -> [w49] mode=indexing
        shift-right: [w50] -> w38
        shift-left: w39 -> [w51]
        tunnel: w37 -> [w44]
        shift-right: [w45] -> w35
        shift-left: w36 -> [w46]
        tunnel: [w42] -> w34 mode=indexing if=w41
        i -> [w43]
        n11 = Equal?(x=w49, y=1) -> (x = y?=w47:bool)
        n12 = case shown="True" w47 {
          selector: w47 -> [w52 _]
          tunnel: w49 -> [_ w66]
          tunnel: w51 -> [w54 w65]
          tunnel: [w54 w64] -> w50
          tunnel: w43 -> [_ w63]
          tunnel: w44 -> [_ w62]
          tunnel: w46 -> [w53 w58]
          tunnel: [w53 w57] -> w45
          tunnel: [w52 w55] -> w41
          frame False {
          }
          frame True {
            n13 = for {
              N: 9 -> [_]
              tunnel: w66 -> [_]
              shift-right: [w79] -> w64
              shift-left: w65 -> [w79]
              tunnel: w63 -> [w72]
              tunnel: w62 -> [w76]
              tunnel: [w68] -> w61 mode=indexing
              i -> [w78]
              n14 = Quotient & Remainder(x=w78, y=3) -> (x-y*floor(x/y)=w71:i32, floor(x/y)=w75:i32)
              n15 = Add(x=w76, y=w75) -> (x+y=w74:i32)
              n16 = Add(x=w72, y=w71) -> (x+y=w70:i32)
              n17 = Decrement(x=w74) -> (x-1=w73:i32)
              n18 = Decrement(x=w70) -> (x-1=w69:i32)
              n19 = Index Array(array=w79, index (row)=w73, index (col)=w69) -> (element=w68:i32)
            }
            "Array 2" <- w61
            n20 = Add Array Elements(numeric array=w61) -> (sum=w60:i32)
            n21 = Increment(x=w58) -> (x+1=w56:i32)
            n22 = Less?(x=w60, y=5) -> (x < y?=w55:bool)
            n23 = Select(t=w56, s=w55, f=w58) -> (s? t:f=w57:i32)
          }
        }
        n24 = Build Array(w44, w43) -> (w42:i32[])
      }
    }
    "Result" <- w24
    "Array 3" <- w25
    n25 = Array Size(array=w25) -> (size(s)=w23:i32[])
    n26 = for {
      tunnel: w25 -> [w29] mode=indexing
      shift-right: [w30] -> w20
      shift-left: w26 -> [w31]
      n27 = call "Replace Array Element__ogtk.vi"("New Element"=0 ("y"), "Indices (>=1D)"=w29, "MultiD Array"=w31) -> ("VMultiD Array"=w32:variant)  [unwired: 7 in, 1 out]
      n28 = Variant To Data(type=w31, Variant=w32) -> (data=w30:i32[][])  [unwired: 1 in, 1 out]
    }
    "Intensity Graph" <- w20
    n29 = Equal?(x=w23, y=i32[] [0, 0]) -> (x = y?=w21:bool)
  }
